vi "X Scale Flipped Write.vi"(4 "error in (no error)":errorcluster, 5 "Value":bool, 6 "Container State":T3, 7 "Display State In":T1) -> (0 "error out":errorcluster, 3 "Display State Out":T1)   [LabVIEW 2017, in "XY Plot Matrix.xctl"]
uses:
  <vilib>/Math Plots/2D Math Plots/XY Plot Matrix/XY Plot Matrix XCtrl/XY Plot Matrix.xctl
  <vilib>/_xctls/Container State.ctl
  <vilib>/Math Plots/2D Math Plots/XY Plot Matrix/XY Plot Matrix XCtrl/State.ctl
  <vilib>/Math Plots/2D Math Plots/XY Plot Matrix/XY Plot Matrix/XY Plot Matrix.lvclass
  e:/builds/penguin/labview/branches/2017/dev/dist/vi.lib/Math Plots/2D Math Plots/2D Plot/2D Plot/2D Plot.lvclass
  <vilib>/Math Plots/2D Math Plots/2D Plot/Action String/XYPlotMatrix Ctrl Act Queue.ctl
  <vilib>/Math Plots/2D Math Plots/2D Plot/Action String/XYPlotMatrix Ctrl Act Cluster.ctl
  <vilib>/Math Plots/2D Math Plots/2D Plot/Action String/2DMathPlot State Class.ctl
  <vilib>/Math Plots/2D Math Plots/2D Plot/2D Plot/2D Plot.lvclass
  <vilib>/_xctls/XControlSupport.lvlib
panel:
  # "Replace the Value Control below with a Control of desired type.\nDo not remove this Control or the others from the connector pane.\nDo not change the connector pane pattern.\nThe Value control should always be the third terminal from top on the input side in the connector pane."
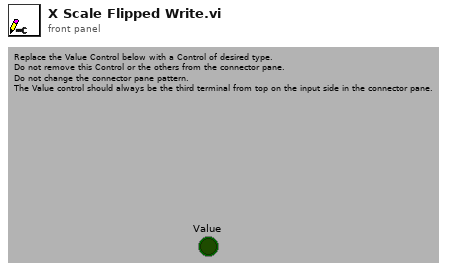
[diagram p1: front panel]
types:
  T1 = typedef "XY Plot Matrix.xctl/State.ctl" = cluster{"XY Plot Matrix.lvclass":refnum<class "XY Plot Matrix.lvclass">, "Control Ref Queue":T2, "Main Frame Color":u32}
  T2 = typedef "XYPlotMatrix Ctrl Act Queue.ctl" = refnum<queue>
  T3 = typedef "XControlSupport.lvlib/Container State.ctl" = cluster{"Indicator?":bool, "Run Mode?":bool, " Refnum":refnum<vi>}
  T4 = typedef "2DMathPlot State Class.ctl" = enum16{"Update All (Undo)", "Update General", "Update Appearance", "Update Format", "Update Scale", "Update Marker", "Update Cursor", "None"}
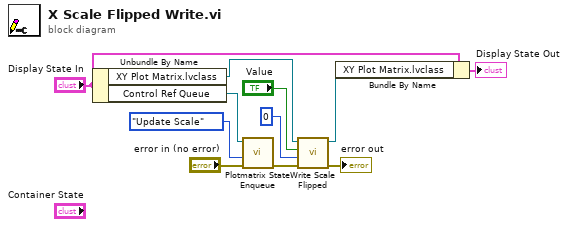
[diagram p0: block diagram]
diagram:
  n1 = Unbundle By Name("Display State In") -> ("XY Plot Matrix.lvclass"=w11:refnum<class "XY Plot Matrix.lvclass">, "Control Ref Queue"=w3:T2)
  n2 = call <vilib>:"Plotmatrix State Enqueue.vi"("error in (no error)"="error in (no error)", "Display State Change Class"=2DMathPlot_State_Class."Update Scale", "Control Ref Queue"=w3) -> ("error out"=w1:errorcluster)  [unwired: 8 out]
  n3 = call <vilib>:"Write Scale Flipped.vi"("error in (no error)"=w1, "Index"=0, "Flipped"="Value", "2D Plot.lvclass in"=w11) -> ("error out"=→"error out":errorcluster, "2D Plot.lvclass out"=w10:refnum<class "XY Plot Matrix.lvclass">)  [unwired: 6 out]
  n4 = Bundle By Name(cluster="Display State In", "XY Plot Matrix.lvclass"=w10) -> (→"Display State Out":T1)
